vi "Cal7-GetCalNumbers.vi"(9 "CalString":string, 10 "StringName":string, 11 "EarlierPoints":bool) -> (1 "Array3":dbl[](array[numeric]), 2 "Array0":dbl[](array[numeric]), 3 "Array2":dbl[](array[numeric]), 4 "Array4":dbl[](array[numeric]), 5 "Array1":dbl[](array[numeric]), 6 "Array5":bool[](array[boolean]))   [LabVIEW 2022 SP3]
uses:
  Anemometry Sub Vis/Globals/Calib_global.vi
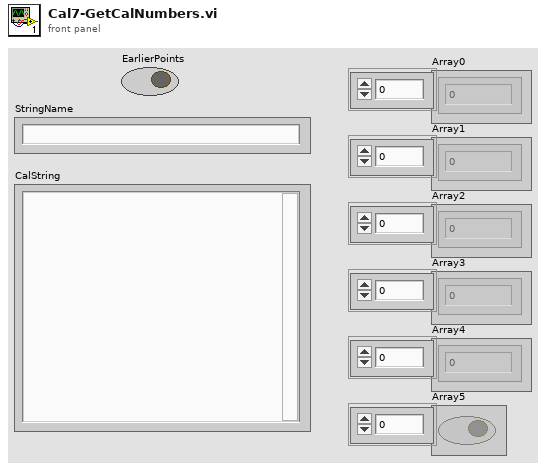
[diagram p1: front panel]
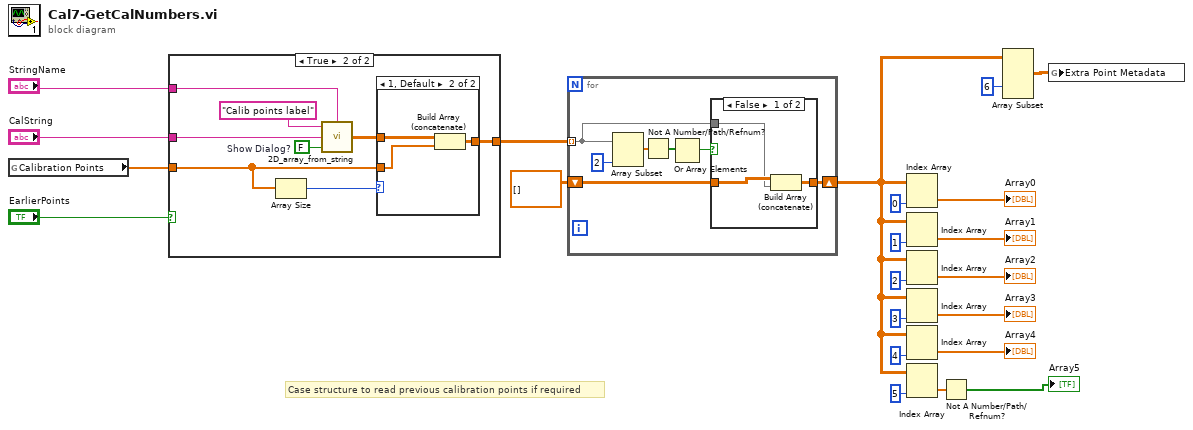
[diagram p0: block diagram]
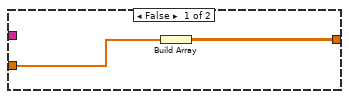
[diagram p3: hidden frame]
diagram:
  # "Case structure to read previous calibration points if required"
  n1 = global read "Calib_global.vi" "Calibration Points"() -> (w19:dbl[])
  n2 = case shown="True" "EarlierPoints" {
    tunnel: "CalString" -> [_ w31]
    tunnel: [w23 w28] -> w20
    tunnel: w19 -> [w24 w27]
    tunnel: "StringName" -> [_ w25]
    frame False {
      n3 = Build Array(w24) -> (w23:dbl[][])
    }
    frame True {
      w30 = FALSE  # Show Dialog?
      n4 = Array Size(array=w27) -> (size(s)=w26:i32)
      n5 = call "2D_array_from_string.vi"("String Name"=w25, "Show Dialog?"=w30, "Input string"=w31, "Array title"="Calib points label") -> ("2D data array"=w29:dbl[][])
      n6 = case shown="1, Default" w26 {
        tunnel: w29 -> [w33 w36]
        tunnel: [w33 w35] -> w28
        tunnel: w27 -> [_ w34]
        frame 0 {
        }
        frame 1, Default {
          n7 = Build Array (concatenate)(w36, w34) -> (w35:dbl[][])
        }
      }
    }
  }
  n8 = for {
    tunnel: w20 -> [w37] mode=indexing
    shift-right: [w38] -> w3
    shift-left: dbl[][] [] -> [w39]
    n9 = Array Subset(array=w37, length=2) -> (w42:dbl[])  [unwired: 1 in]
    n10 = Not A Number/Path/Refnum?(number/path/refnum=w42) -> (NaN/Path/Refnum?=w41:bool[])
    n11 = Or Array Elements(Boolean array=w41) -> (logical OR=w40:bool)
    n12 = case shown="False" w40 {
      tunnel: w39 -> [w46 w47]
      tunnel: w37 -> [w45 _]
      tunnel: [w44 w47] -> w38
      frame False {
        n13 = Build Array (concatenate)(w46, w45) -> (w44:dbl[][])
      }
      frame True {
      }
    }
  }
  n14 = Index Array(array=w3, index (col)=0) -> (element=→"Array0":dbl[])  [unwired: 1 in]
  n15 = Index Array(array=w3, index (col)=1) -> (element=→"Array1":dbl[])  [unwired: 1 in]
  n16 = Index Array(array=w3, index (col)=2) -> (element=→"Array2":dbl[])  [unwired: 1 in]
  n17 = Index Array(array=w3, index (col)=3) -> (element=→"Array3":dbl[])  [unwired: 1 in]
  n18 = Index Array(array=w3, index (col)=4) -> (element=→"Array4":dbl[])  [unwired: 1 in]
  n19 = Index Array(array=w3, index (col)=5) -> (element=w16:dbl[])  [unwired: 1 in]
  n20 = Not A Number/Path/Refnum?(number/path/refnum=w16) -> (NaN/Path/Refnum?=→"Array5":bool[])
  n21 = Array Subset(array=w3, index (col)=6 ("index")) -> (w1:dbl[][])  [unwired: 3 in]
  n22 = global write "Calib_global.vi" "Extra Point Metadata"(w1) -> ()
